vi "Stream Circle On Axis Subset.vi"(4 "Direction (0: clockwise)":u16(ring) items=["clockwise", "counter-clockwise"], 5 "Symbolic Axes":string[](array[string]), 6 "Position Mode (0: absolute)":u16(ring) items=["absolute", "relative"], 7 "Center":i64[](array[numeric]), 8 "error in (no error)":errorcluster, 9 "Device Number":string, 10 "Stream Number (1)":u8=1, 11 "VISA resource name":refnum<visa-resource-name>) -> (0 "error out":errorcluster, 3 "VISA resource name out":refnum<visa-resource-name>)   [LabVIEW 2018, in "Zaber A Series.lvlib"]
doc: "Adds a circle command to an open stream, using a subset of the stream's axes. The position where the previous stream command leaves the device will be a point on the circle. The Center Position input specifies where the center of the circle will be, either in absolute coordinates or relative to the device position; the Position Mode input controls whether it is absolute or relative.\n\nThe center point is specified in microstep units - use the Convert Position to Device Units VI to convert from standard measurements.\n\nThe Symbolic Axes input specifies which of the stream's axes the command will operate on. This should contain two letters as separate array entries. The entries in the Symbolic Axes input are not axes numbers but letters that map to axes in the order the axes were added to the stream. For example, if the stream was set up with axes [1, 3, 2] then the symbol definitions will be a = 1, b = 3, c = 2. You can also permute the order in this input, so if you pass Symbolic Axes the input [c, b] in this example, then the coordinates you give will be for physical axes [2, 3].\n\nCircles are only supported on two axes, so this VI should be used instead of the other Stream Circle VIs if your stream is set up with more than two axes.\n\nThis VI does not check in advance for error conditions such as streams not being supported or the stream not being open.\n\nThis VI requires that the device have Firmware version 7, that the Initialize VI has been called with the same serial port and that the specified stream is open."
uses:
  Zaber A Series.lvlib
  Private/All Commands.ctl
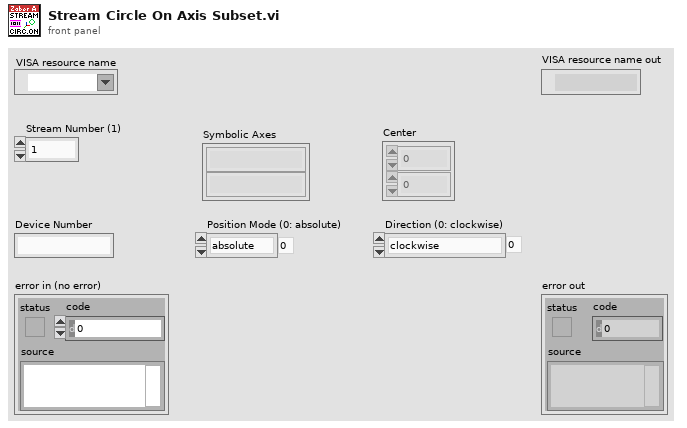
[diagram p1: front panel]
types:
  T1 = typedef "Zaber A Series.lvlib/All Commands.ctl" = string
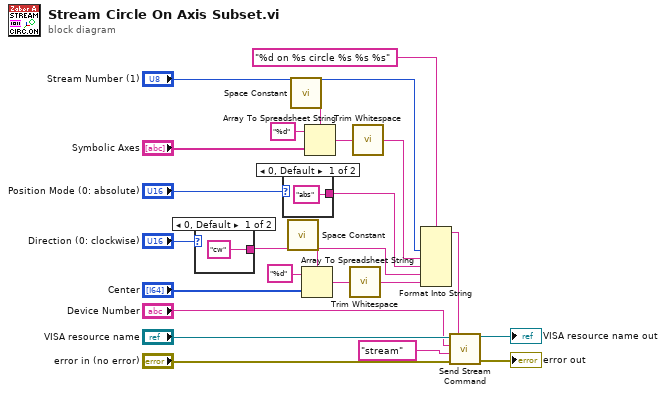
[diagram p0: block diagram]
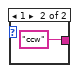
[diagram p2: hidden frame]
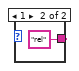
[diagram p3: hidden frame]
diagram:
  n1 = case shown="0, Default" "Direction (0: clockwise)" {
    tunnel: ["cw" "ccw"] -> w7
    frame 0, Default {
    }
    frame 1 {
    }
  }
  n2 = case shown="0, Default" "Position Mode (0: absolute)" {
    tunnel: ["abs" "rel"] -> w6
    frame 0, Default {
    }
    frame 1 {
    }
  }
  n3 = call <vilib>:"Space Constant.vi"() -> ("String"=w11:string)
  n4 = call <vilib>:"Space Constant.vi"() -> ("String"=w4:string)
  n5 = Array To Spreadsheet String(delimiter (Tab)=w11, array="Center", 3:"%d" ("format string")) -> (spreadsheet string=w14:string)
  n6 = Array To Spreadsheet String(delimiter (Tab)=w4, array="Symbolic Axes", 3:"%d" ("format string")) -> (spreadsheet string=w5:string)
  n7 = call <vilib>:"Trim Whitespace.vi"("string"=w14) -> ("trimmed string"=w8:string)  [unwired: 1 in]
  n8 = call <vilib>:"Trim Whitespace.vi"("string"=w5) -> ("trimmed string"=w2:string)  [unwired: 1 in]
  n9 = Format Into String(format string="%d on %s circle %s %s %s", "Stream Number (1)", w2, w6, w7, w8) -> (resulting string=w10:string)  [unwired: 2 in, 1 out]
  n10 = call "Send Stream Command.vi"("Data"=w10, "error in (no error)"="error in (no error)", "Command"=T1 "stream" ("Complete Command List"), "Device Number"="Device Number", "VISA resource name"="VISA resource name") -> ("error out"=→"error out":errorcluster, "VISA resource name out"=→"VISA resource name out":refnum<visa-resource-name>)  [unwired: 5 in]
